vi "Write Verbose.vi"(10 "Verbose":bool, 11 "Test Runner in":refnum<class "Test Runner.lvclass">) -> (3 "Test Runner out":refnum<class "Test Runner.lvclass">)   [LabVIEW 2013, in "Caraya.lvlib" / "Test Runner.lvclass"]
uses:
  Test Runner.lvclass
  Test Runner.lvclass/Test Runner.ctl
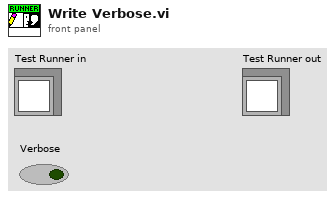
[diagram p1: front panel]
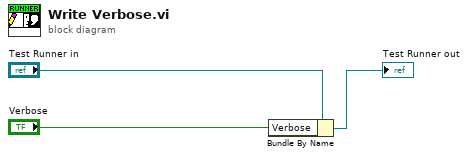
[diagram p0: block diagram]
diagram:
  n1 = Bundle By Name(cluster="Test Runner in", "Verbose"="Verbose") -> (→"Test Runner out":refnum<class "Test Runner.lvclass">)
